vi "Load TSP File.vi"() -> (0 "DIMENSION":i32, 1 "Distance Opt":dbl, 2 "Tour Selection":i32[](array[numeric]), 3 "Coordinate[]":T1[](array[typedef]))   [LabVIEW 2015, in "TSP Library.lvlib"]
uses:
  TSP Library.lvlib
  TypeDef/Coordinate.ctl
panel:
  out "City's":cluster{"X":dbl, "Y":dbl}[](graph)
  in  "Exit":bool
  in  "Load Data":bool
  out "DIMENSION Opt":i32
  out "SizeOpt IsOk":bool
  out "ParseOpt Size":i32
  in  "Opt File Path":path
  out "Parse Size":i32
  out "Size IsOk":bool
  in  "TSP File Path":path
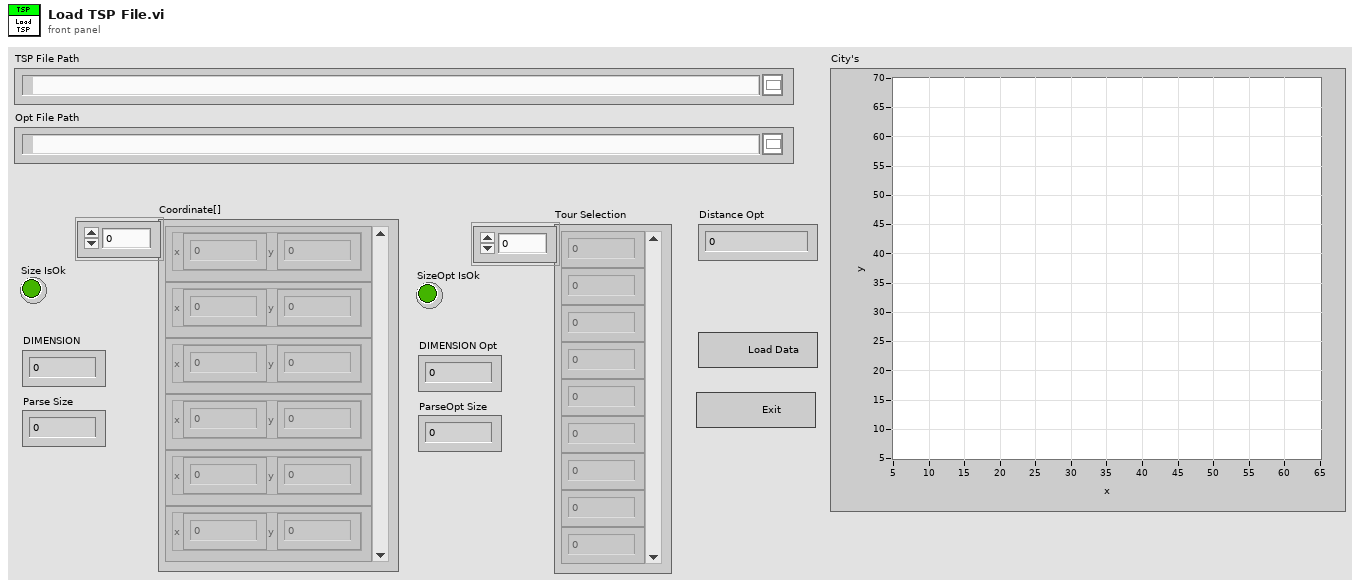
[diagram p1: front panel]
types:
  T1 = typedef "TSP Library.lvlib/Coordinate.ctl" = cluster{"x":dbl, "y":dbl}
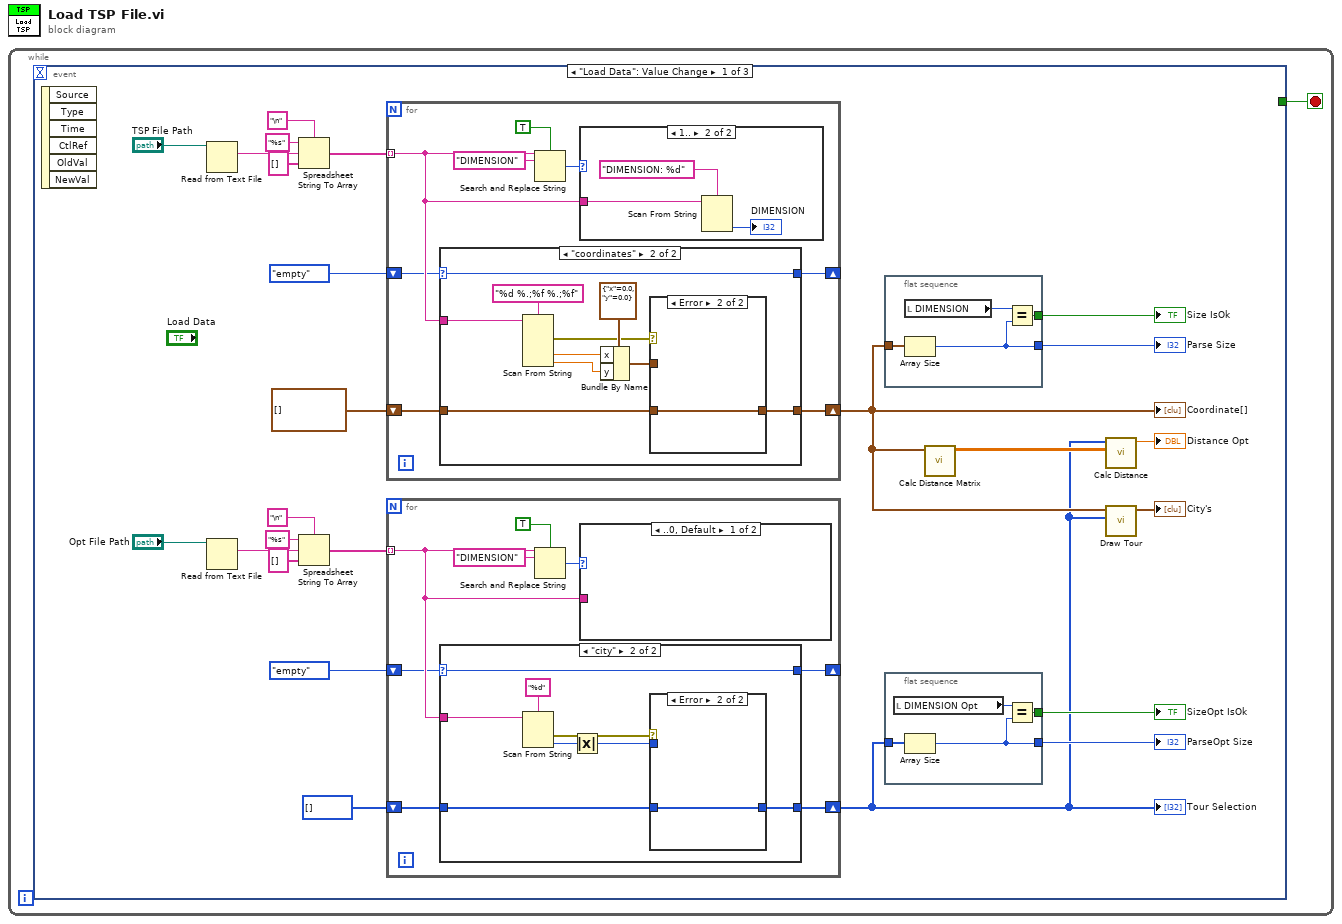
[diagram p0: block diagram]
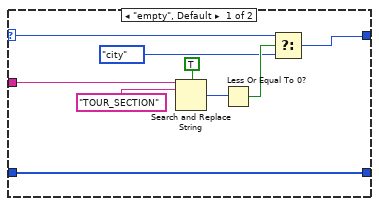
[diagram p2: hidden frame]
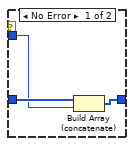
[diagram p3: hidden frame]
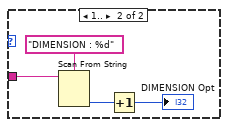
[diagram p4: hidden frame]
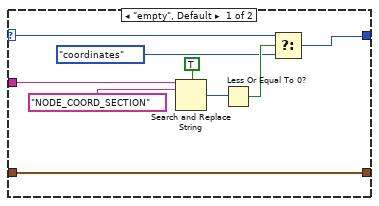
[diagram p5: hidden frame]
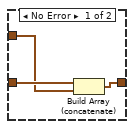
[diagram p6: hidden frame]
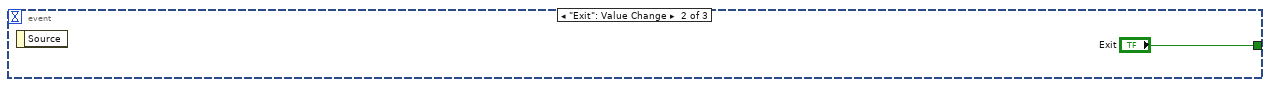
[diagram p8: hidden frame]
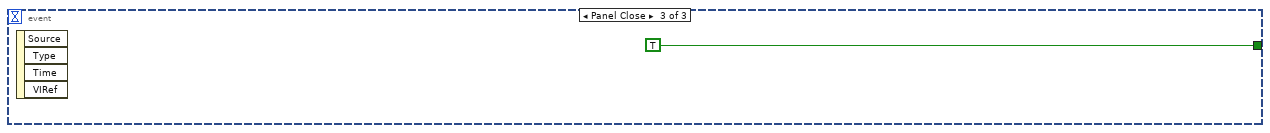
[diagram p9: hidden frame]
diagram:
  n1 = while {
    stop <- w1 stop-if-true
    n2 = event shown="[0] \"Load Data\": Value Change" {
      selector: _ -> [_ _ _]
      dyn-events: _ -> [_ _ _]
      timeout: _ -> [_ _ _]
      tunnel: [_ "Exit" TRUE ("Exit")] -> w1
      event "Load Data": Value Change {
        n3 = event-data() -> ()  [unwired: 1 in, 6 out]
        n4 = Read from Text File(file (use dialog)="TSP File Path") -> (text=w25:string)  [unwired: 3 in, 3 out]
        n5 = Read from Text File(file (use dialog)="Opt File Path") -> (text=w8:string)  [unwired: 3 in, 3 out]
        n6 = Spreadsheet String To Array(delimiter (Tab)="\n", format string="%s", spreadsheet string=w25, array type (2D Dbl)=string[] []) -> (array=w21:string[])
        n7 = Spreadsheet String To Array(delimiter (Tab)="\n", format string="%s", spreadsheet string=w8, array type (2D Dbl)=string[] []) -> (array=w12:string[])
        n8 = for {
          tunnel: w21 -> [w72] mode=indexing
          shift-right: [w70] -> _
          shift-left: enum16{"empty", "coordinates"}."empty" -> [w71]
          shift-right: [w68] -> w4
          shift-left: T1[] [] ("Array") -> [w69]
          n9 = case shown="\"coordinates\"" w71 {
            selector: w71 -> [w79 w94]
            tunnel: w72 -> [w82 w93]
            tunnel: [w78 w94] -> w70
            tunnel: w69 -> [w76 w87]
            tunnel: [w76 w86] -> w68
            frame "empty", Default {
              n10 = Search and Replace String(case sensitive?=TRUE ("ignore case? (F)"), input string=w82, search string="NODE_COORD_SECTION") -> (number of replacements=w81:i32)  [unwired: 5 in, 3 out]
              n11 = Less Or Equal To 0?(x=w81) -> (x <= 0?=w80:bool)
              n12 = Select(t=w79, s=w80, f=enum16{"empty", "coordinates"}."coordinates") -> (s? t:f=w78:enum16{"empty", "coordinates"})
            }
            frame "coordinates" {
              n13 = Scan From String(format string="%d %.;%f %.;%f", input string=w93) -> (error out=w88:errorcluster, output 2=w90:dbl, output 3=w89:dbl)  [unwired: 6 in, 2 out]
              n14 = Bundle By Name(cluster=T1 {"x"=0.0, "y"=0.0} ("Coordinate"), "x"=w90, "y"=w89) -> (w85:T1)
              n15 = case shown="Error" w88 {
                tunnel: [w96 w98] -> w86
                tunnel: w87 -> [w97 w98]
                tunnel: w85 -> [w95 _]
                frame No Error {
                  n16 = Build Array (concatenate)(w97, w95) -> (w96:T1[])
                }
                frame Error {
                }
              }
            }
          }
          n17 = Search and Replace String(case sensitive?=TRUE ("ignore case? (F)"), input string=w72, search string="DIMENSION") -> (number of replacements=w73:i32)  [unwired: 5 in, 3 out]
          n18 = case shown="1.." w73 {
            tunnel: w72 -> [_ w101]
            frame ..0, Default {
            }
            frame 1.. {
              n19 = Scan From String(format string="DIMENSION: %d", input string=w101) -> (output 1=→"DIMENSION":i32)  [unwired: 3 in, 3 out]
            }
          }
        }
        "Coordinate[]" <- w4
        n20 = for {
          tunnel: w12 -> [w35] mode=indexing
          shift-right: [w33] -> _
          shift-left: enum16{"empty", "city"}."empty" -> [w34]
          shift-right: [w31] -> w3
          shift-left: i32[] [] ("Array") -> [w32]
          n21 = case shown="\"city\"" w34 {
            selector: w34 -> [w42 w55]
            tunnel: w35 -> [w45 w54]
            tunnel: [w41 w55] -> w33
            tunnel: w32 -> [w39 w51]
            tunnel: [w39 w50] -> w31
            frame "empty", Default {
              n22 = Search and Replace String(case sensitive?=TRUE ("ignore case? (F)"), input string=w45, search string="TOUR_SECTION") -> (number of replacements=w44:i32)  [unwired: 5 in, 3 out]
              n23 = Less Or Equal To 0?(x=w44) -> (x <= 0?=w43:bool)
              n24 = Select(t=w42, s=w43, f=enum16{"empty", "city"}."city") -> (s? t:f=w41:enum16{"empty", "city"})
            }
            frame "city" {
              n25 = Scan From String(format string="%d", input string=w54) -> (error out=w52:errorcluster, output 1=w49:i32)  [unwired: 3 in, 2 out]
              n26 = Absolute Value(x=w49) -> (abs(x)=w48:i32)
              n27 = case shown="Error" w52 {
                tunnel: [w57 w59] -> w50
                tunnel: w51 -> [w58 w59]
                tunnel: w48 -> [w56 _]
                frame No Error {
                  n28 = Build Array (concatenate)(w58, w56) -> (w57:i32[])
                }
                frame Error {
                }
              }
            }
          }
          n29 = Search and Replace String(case sensitive?=TRUE ("ignore case? (F)"), input string=w35, search string="DIMENSION") -> (number of replacements=w36:i32)  [unwired: 5 in, 3 out]
          n30 = case shown="..0, Default" w36 {
            tunnel: w35 -> [_ w63]
            frame ..0, Default {
            }
            frame 1.. {
              n31 = Scan From String(format string="DIMENSION : %d", input string=w63) -> (output 1=w61:i32)  [unwired: 3 in, 3 out]
              n32 = Increment(x=w61) -> (x+1=→"DIMENSION Opt":i32)
            }
          }
        }
        "Tour Selection" <- w3
        n33 = flat-sequence {
          tunnel: w4 -> [w67]
          tunnel: [w65] -> w18
          tunnel: [w64] -> w17
          frame #0 {
            n34 = local read "DIMENSION"() -> (w66:i32)
            n35 = Array Size(array=w67) -> (size(s)=w64:i32)
            n36 = Equal?(x=w66, y=w64) -> (x = y?=w65:bool)
          }
        }
        n37 = flat-sequence {
          tunnel: w3 -> [w30]
          tunnel: [w28] -> w15
          tunnel: [w27] -> w16
          frame #0 {
            n38 = local read "DIMENSION Opt"() -> (w29:i32)
            n39 = Array Size(array=w30) -> (size(s)=w27:i32)
            n40 = Equal?(x=w29, y=w27) -> (x = y?=w28:bool)
          }
        }
        n41 = call "Calc Distance Matrix.vi"("Coordinate[]"=w4) -> ("Distance Matrix"=w5:dbl[][])  [unwired: 10 in]
        n42 = call "Calc Distance.vi"("Distance Matrix"=w5, "Tour"=w3) -> ("Distance"=→"Distance Opt":dbl)  [unwired: 9 in]
        n43 = call "Draw Tour.vi"("Tour"=w3, "Coordinate[]"=w4) -> ("City's"=→"City's":cluster{"X":dbl, "Y":dbl}[])  [unwired: 9 in]
        "Size IsOk" <- w18
        "Parse Size" <- w17
        "SizeOpt IsOk" <- w15
        "ParseOpt Size" <- w16
      }
      event "Exit": Value Change {
        n44 = event-data() -> ()  [unwired: 1 in, 1 out]
      }
      event Panel Close {
        n45 = event-data() -> ()  [unwired: 1 in, 4 out]
      }
    }
  }
